vi "S2C_VLFT10_Proc_GlobalSensorScales.vi"(8 "Error In":errorcluster, 11 "Scales":string) -> (0 "Error Out":errorcluster, 3 "Result":string)   [LabVIEW 2015]
uses:
  Fornax/VIs/S2C_FORNAX_Proc_Globals.vi
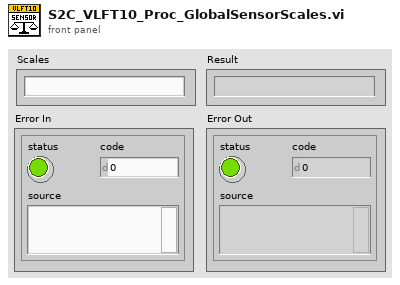
[diagram p1: front panel]
types:
  T1 = cluster{"ScaleType":u16, "ScaleAction":u16, "PreDelay (ms)":i32, "PostDelay (ms)":i32, "ClearFornaxMsgs":bool}
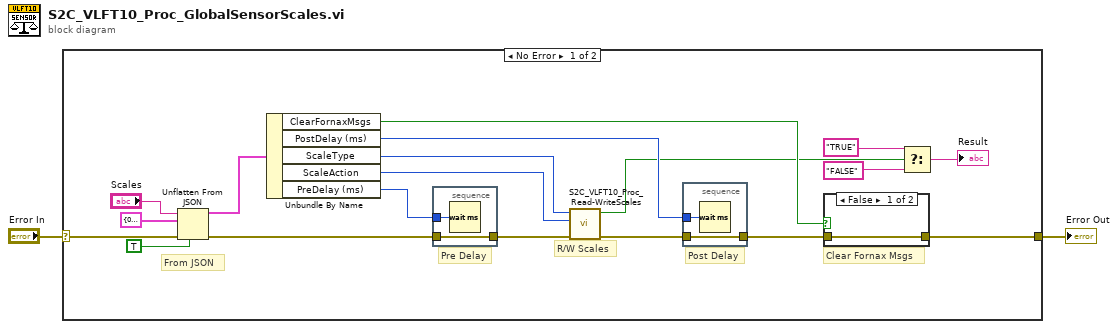
[diagram p0: block diagram]
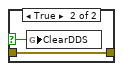
[diagram p2: hidden frame]
diagram:
  n1 = case shown="No Error" "Error In" {
    selector: "Error In" -> [w19 w29]
    tunnel: [w17 w29] -> w1
    frame No Error {
      # "R/W Scales"
      # "Clear Fornax Msgs"
      # "Post Delay"
      # "Pre Delay"
      # "From JSON"
      n2 = Unflatten From JSON(JSON string="Scales", type and defaults=T1 {"ScaleType"=0, "ScaleAction"=0, "PreDelay (ms)"=0, "PostDelay (ms)"=0, "ClearFornaxMsgs"=FALSE}, default null elements? (F)=TRUE, error in (no error)=w19) -> (value=w16:T1, error out=w18:errorcluster)  [unwired: 3 in]
      n3 = Unbundle By Name(w16) -> ("ClearFornaxMsgs"=w10:bool, "PostDelay (ms)"=w14:i32, "ScaleType"=w11:u16, "ScaleAction"=w13:u16, "PreDelay (ms)"=w12:i32)
      n4 = stacked-sequence {
        tunnel: w18 -> [w28]
        tunnel: [w28] -> w9
        tunnel: w12 -> [w27]
        frame #0 {
          n5 = Wait (ms)(milliseconds to wait=w27) -> ()  [unwired: 1 out]
        }
      }
      n6 = call "S2C_VLFT10_Proc_Read-WriteScales.vi"("Error In"=w9, "ScaleAction"=w13, "ScaleType"=w11) -> ("Error Out"=w8:errorcluster, "Pass?"=w6:bool)  [unwired: 7 in]
      n7 = stacked-sequence {
        tunnel: w8 -> [w26]
        tunnel: [w26] -> w7
        tunnel: w14 -> [w25]
        frame #0 {
          n8 = Wait (ms)(milliseconds to wait=w25) -> ()  [unwired: 1 out]
        }
      }
      n9 = case shown="False" w10 {
        selector: w10 -> [_ w23]
        tunnel: w7 -> [w22 w24]
        tunnel: [w22 w24] -> w17
        frame False {
        }
        frame True {
          n10 = global write "S2C_FORNAX_Proc_Globals.vi" "ClearDDS"(w23) -> ()
        }
      }
      n11 = Select(t="TRUE", s=w6, f="FALSE") -> (s? t:f=→"Result":string)
    }
    frame Error {
    }
  }
  "Error Out" <- w1
